vi "ValiseMarlin.vi"() -> ()   [LabVIEW 2017]
uses:
  Globals/VarGlobUIStopLoops.vi
  <resource>/objmgr/daqmx.rc
  DefDeType/WhichPath.ctl
  <vilib>/DAQmx/write.llb/DAQmx Write (Digital Bool 1Line 1Point).vi
  <vilib>/DAQmx/create/channels.llb/DAQmx Create Channel (DO-Digital Output).vi
  DefDeType/ClusterRefCtrl.ctl
panel:
  in  "Reprocess":bool
  in  "Next Test":u32
  out "AcqTime(s)":u16(slide) scale=0.0..1000.0
  out "Recording":bool
  in  "EnregistrerPtEtal":bool
  out "Projet":string
  in  "Essais réalisés":i32(listbox)
  out "Reload Config":bool
  out "EntreesTensions":dbl[][](graph)
  in  "ChangerConfig":bool
  out "iterationMonitoringLoop":i32
  out "iterationEventLoop":i32
  in  "Instruction":u8
  in  "Stop Enreg.":bool
  in  "Enregistrer":bool
  out "EtatValise":string
  out "AmplisPonts":dbl[][](graph)
  in  "Quitter":bool
  # "Commandes"
  # "Entrées Pont de Wheastone"
  # "Essais Réalisés"
  # "Entrées Tensions"
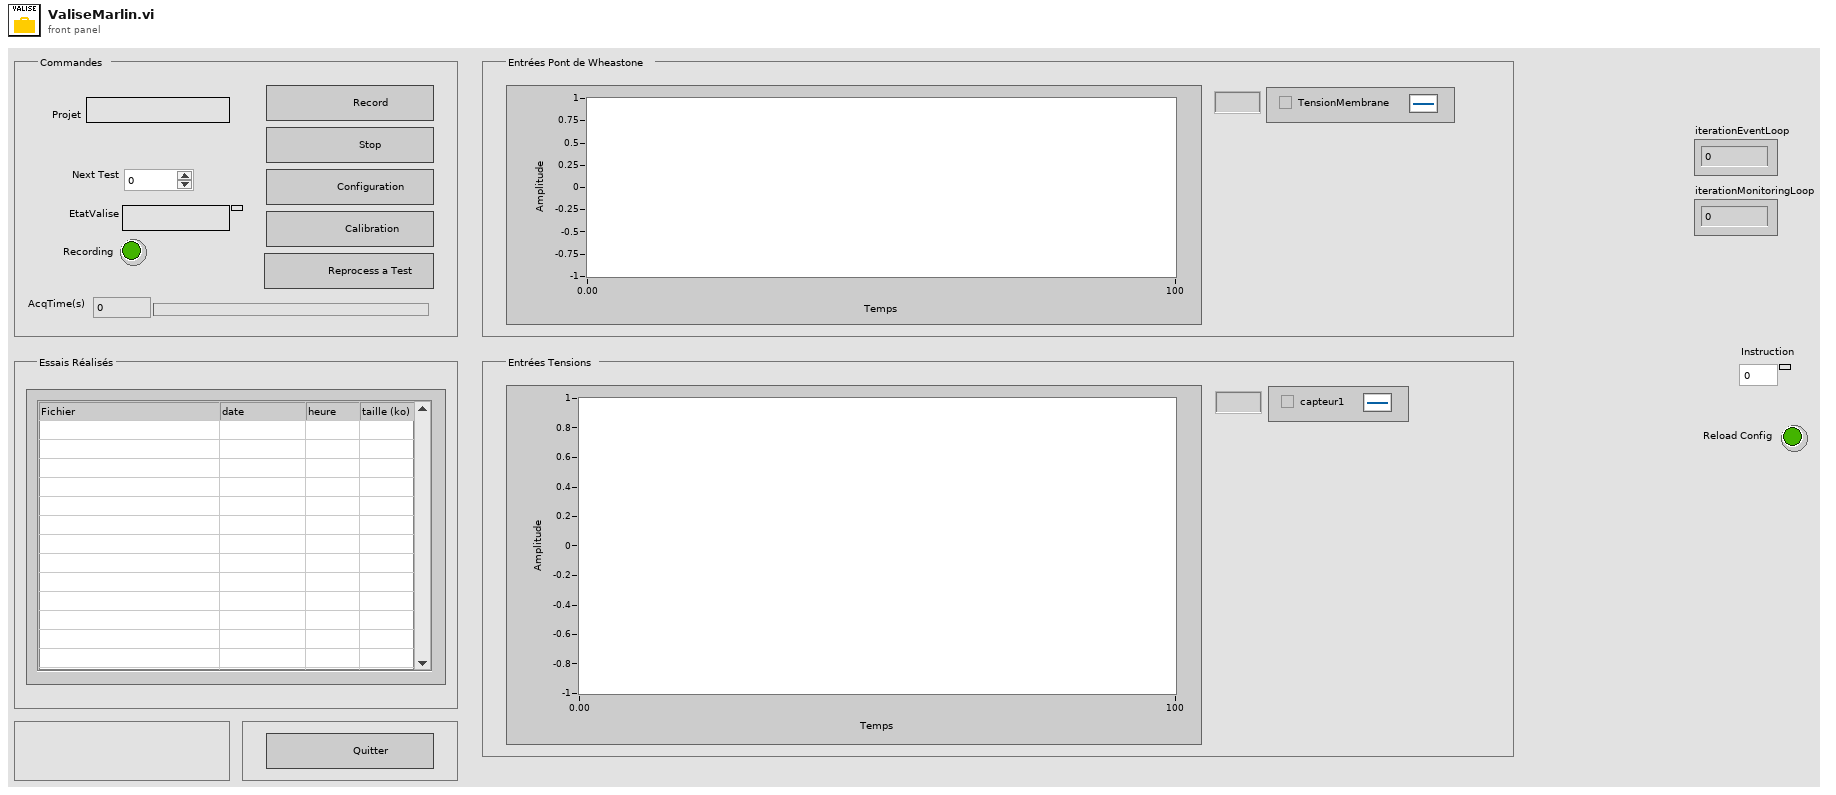
[diagram p1: front panel]
types:
  T1 = enum8{"Enabled", "Disabled", "Disabled and Grayed Out"}
  T2 = typedef "ClusterRefCtrl.ctl" = cluster{"Essais réalisés":refnum<vi>, "EnregistrerPtEtal":refnum<vi>, "ChangerConfig":refnum<vi>, "Enregistrer":refnum<vi>, "Reprocess":refnum<vi>}
  T3 = enum32{"Invalid", "Standard", "Closed", "Hidden", "Minimized", "Maximized"}
  T4 = cluster{"AcqTime(s)":refnum<vi>, "EntreesTensions":refnum<vi>, "AmplisPonts":refnum<vi>}
  T5 = typedef "ConfigTotale.ctl" = cluster{"VoltageChannels":T6, "WheastoneBridgeChannels":T7, "Configuration":T8}
  T6 = typedef "VoltageChannels.ctl" = cluster{"ChannelNames":string[], "Sensitivity(Unit/V)":dbl[], "AutoZero":bool[], "ChannelUnits":string[], "Offsets(Units)":dbl[], "Graph Num":u8[]}
  T7 = typedef "WBridgeChannels.ctl" = cluster{"ChannelNames":string[], "Sensitivity(Unit/V)":dbl[], "AutoZero":bool[], "ChannelUnits":string[], "Offsets(Units)":dbl[], "Graph Num":u8[]}
  T8 = typedef "Configuration.ctl" = cluster{"AcqSamplingRate(Hz)":u32, "AcqTime(s)":u32, "Trigger":bool, "NbVoltageChannels":u32, "NbWBridgeChannels":u32, "Qualisys":bool, "Hexapode":bool, "FinalSamplingRate(Hz)":u32, "QualisysDataType":enum16{"6DOF", "3DTracking", "6DOF + 3D"}, "Nortek":bool, "HBM":bool}
  T9 = typedef "WhichPath.ctl" = enum16{"DossierProjet", "Config", "Meas", "MeasPCI", "MeasCRIO1", "MeasCRIO2", "MeasQualisys", "MeasHBM", "MeasTDMS", "Fig", "Res"}
  T10 = typedef "MergeFileConfig.ctl" = cluster{"Test Num : ":u32, "Project :":string, "Qualisys file":path, "HBM file":path, "QualisysDataType":enum16{"6DOF", "3DTracking", "6DOF + 3D"}, "Qualisys":bool, "HBM":bool}
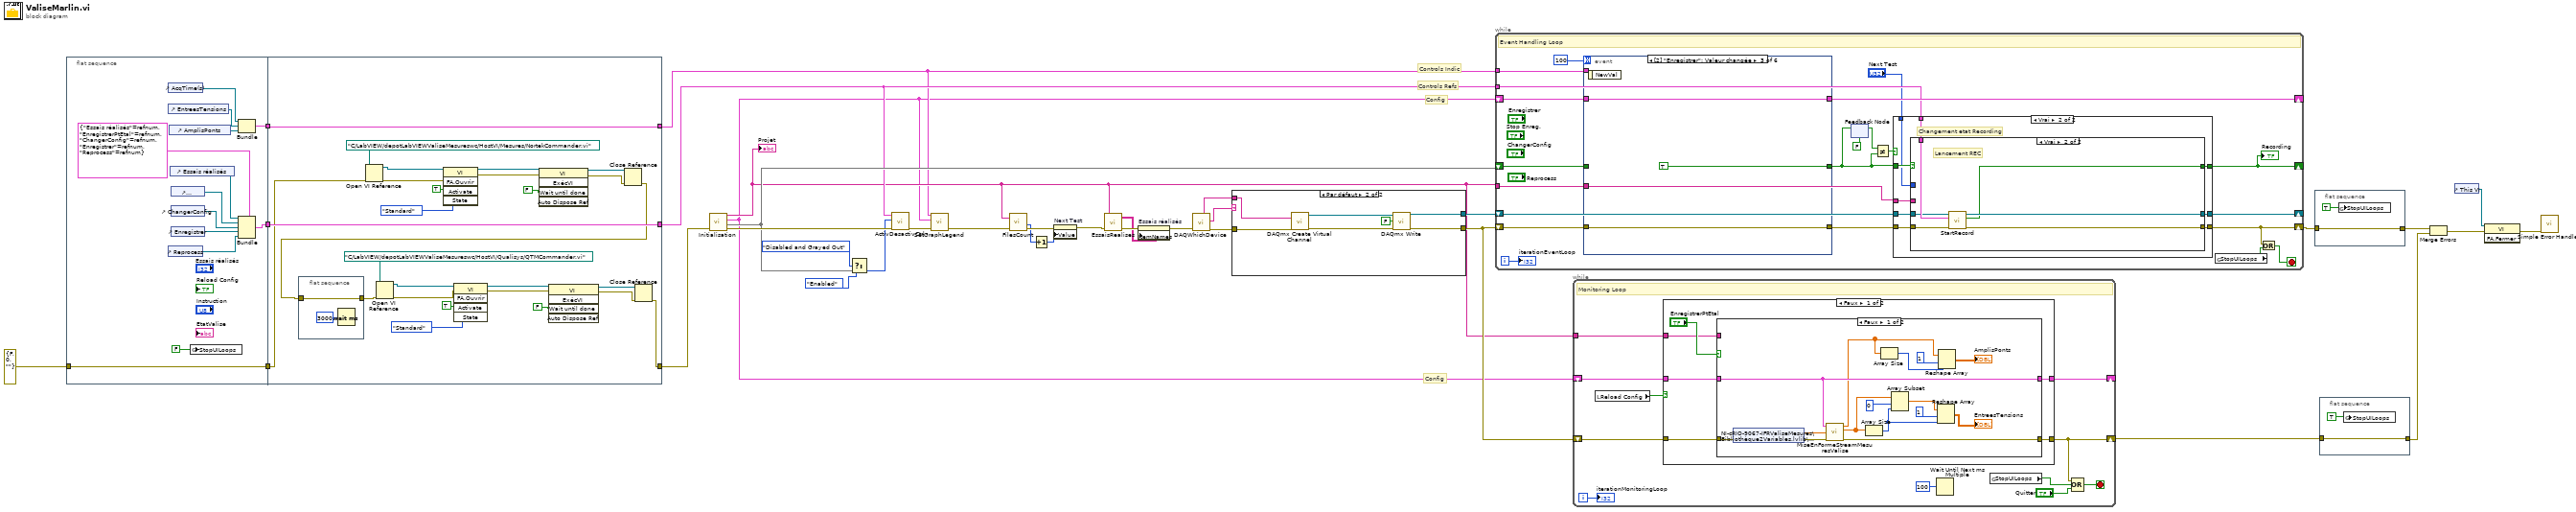
[diagram p0: block diagram]
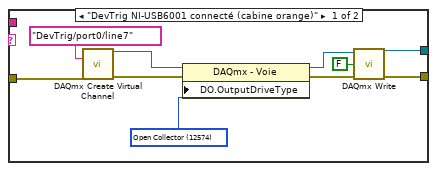
[diagram p2: hidden frame]
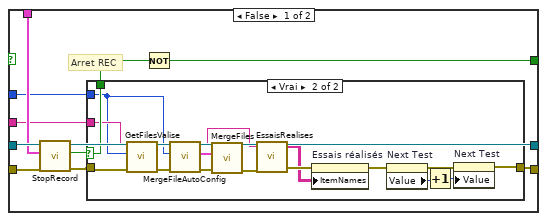
[diagram p4: hidden frame]
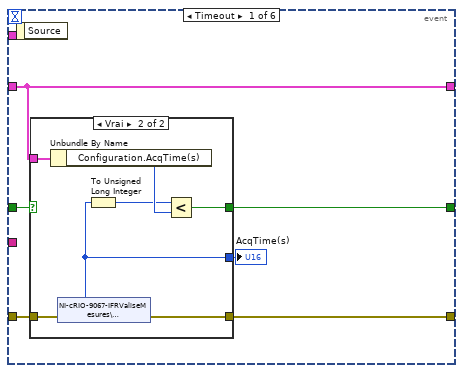
[diagram p6: hidden frame]
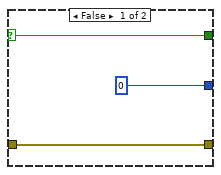
[diagram p7: hidden frame]
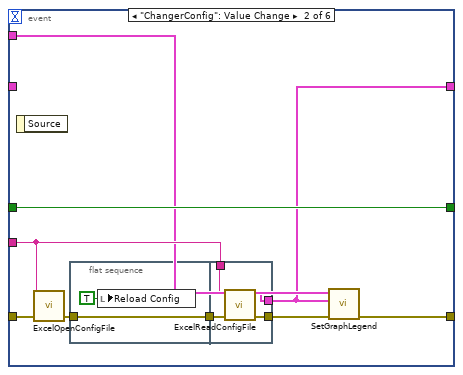
[diagram p8: hidden frame]
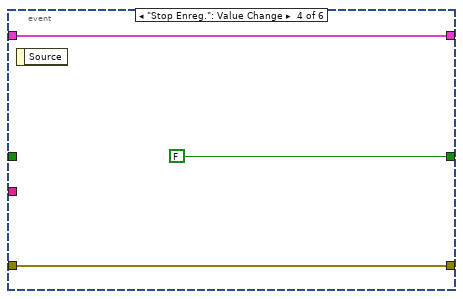
[diagram p9: hidden frame]
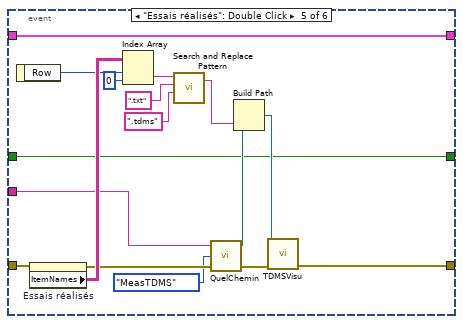
[diagram p10: hidden frame]
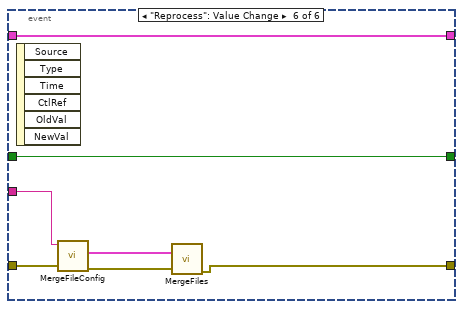
[diagram p11: hidden frame]
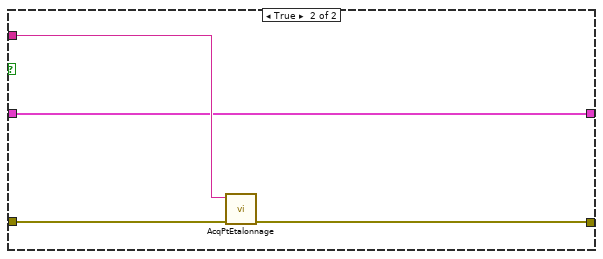
[diagram p12: hidden frame]
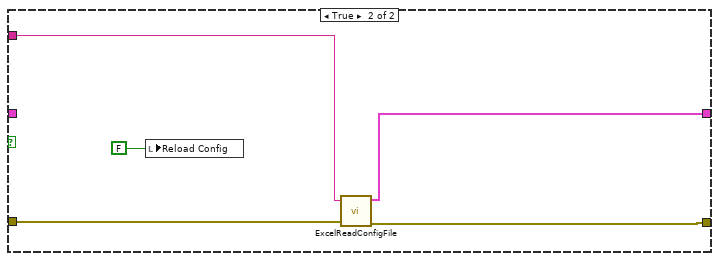
[diagram p13: hidden frame]
diagram:
  # "Controls Indic"
  # "Config"
  # "Config"
  # "Controls Refs"
  n1 = flat-sequence {
    tunnel: errorcluster {"status"=FALSE, "code"=0, "source"=""} ("entrée d'erreur (pas d'erreur)") -> [w47]
    tunnel: [w47] -> w3
    tunnel: [w42] -> w2
    tunnel: [w38] -> w1
    tunnel: [w73] -> w14
    tunnel: [w74] -> w21
    tunnel: [w51] -> w4
    tunnel: w3 -> [w52]
    tunnel: w2 -> [w74]
    tunnel: w1 -> [w73]
    frame #0 {
      n2 = control-ref of="EntreesTensions"() -> (w40:refnum<vi>)
      n3 = control-ref of="AcqTime(s)"() -> (w39:refnum<vi>)
      n4 = control-ref of="Reprocess"() -> (w36:refnum<vi>)
      n5 = control-ref of="AmplisPonts"() -> (w41:refnum<vi>)
      n6 = control-ref of="Essais réalisés"() -> (w43:refnum<vi>)
      n7 = control-ref of="EnregistrerPtEtal"() -> (w44:refnum<vi>)
      n8 = control-ref of="ChangerConfig"() -> (w45:refnum<vi>)
      n9 = control-ref of="Enregistrer"() -> (w46:refnum<vi>)
      n10 = global write "VarGlobUIStopLoops.vi" "StopUILoops"(FALSE ("StopUILoops")) -> ()
      n11 = Bundle("AcqTime(s)"=w39, "EntreesTensions"=w40, "AmplisPonts"=w41) -> (w38:T4)  [unwired: 1 in]
      n12 = Bundle(cluster=T2 {"Essais réalisés"=refnum, "EnregistrerPtEtal"=refnum, "ChangerConfig"=refnum, "Enregistrer"=refnum, "Reprocess"=refnum} ("Cluster"), "Essais réalisés"=w43, "EnregistrerPtEtal"=w44, "ChangerConfig"=w45, "Enregistrer"=w46, "Reprocess"=w36) -> (w42:T2)
    }
    frame #1 {
      n13 = flat-sequence {
        tunnel: w50 -> [w76]
        tunnel: [w76] -> w49
        frame #0 {
          n14 = Wait (ms)(milliseconds to wait=u32 3000) -> ()  [unwired: 1 out]
        }
      }
      n15 = Open VI Reference(vi path=path "C:/LabVIEW/depotLabVIEWValiseMesureswc/HostVI/Mesures/NortekCommander.vi", error in (no error)=w52) -> (vi reference=w54:refnum<vi>, error out=w55:errorcluster)  [unwired: 4 in]
      n16 = Open VI Reference(vi path=path "C:/LabVIEW/depotLabVIEWValiseMesureswc/HostVI/Qualisys/QTMCommander.vi", error in (no error)=w49) -> (vi reference=w71:refnum<vi>, error out=w70:errorcluster)  [unwired: 4 in]
      n17 = invoke class="VI" method="FA.Ouvrir"(reference=w54, error in=w55, "Activate"=TRUE ("Activate?"), "State"=T3."Standard") -> (reference out=w57:refnum<vi>, error out=w56:errorcluster)  [unwired: 1 in, 3 out]
      n18 = invoke class="VI" method="FA.Ouvrir"(reference=w71, error in=w70, "Activate"=TRUE ("Activate?"), "State"=T3."Standard") -> (reference out=w68:refnum<vi>, error out=w69:errorcluster)  [unwired: 1 in, 3 out]
      n19 = invoke class="VI" method="ExécVI"(reference=w57, error in=w56, "Wait until done"=FALSE ("Wait Until Done")) -> (reference out=w58:refnum<vi>, error out=w59:errorcluster)  [unwired: 2 in, 3 out]
      n20 = invoke class="VI" method="ExécVI"(reference=w68, error in=w69, "Wait until done"=FALSE ("Wait Until Done")) -> (reference out=w67:refnum<vi>, error out=w66:errorcluster)  [unwired: 2 in, 3 out]
      n21 = Close Reference(reference=w58, error in (no error)=w59) -> (error out=w50:errorcluster)
      n22 = Close Reference(reference=w67, error in (no error)=w66) -> (error out=w51:errorcluster)
    }
  }
  n23 = call "Initialisation.vi"("Error In"=w4) -> ("Error Out"=w26:errorcluster, 1:w25, "ConfigurationTotale"=w13:T5, "NomProjetOUT"=w20:string)  [unwired: 3 in]
  "Projet" <- w20
  n24 = Select(t=T1."Disabled and Grayed Out" ("Disabled"), s=w25, f=T1."Enabled" ("Disabled")) -> (s? t:f=w22:T1)
  n25 = call "ActivDesactivCtrl.vi"("error in (no error)"=w26, "Disabled"=w22, "Cluster"=w21) -> ("error out"=w15:errorcluster)  [unwired: 4 in]
  n26 = call "SetGraphLegend.vi"("error in (no error)"=w15, "ConfigTotale"=w13, "ClusterRefGraphs"=w14) -> ("error out"=w12:errorcluster)  [unwired: 4 in]
  n27 = call "FilesCount.vi"("NomProjet"=w20, "entrée d'erreur"=w12) -> ("NextTestNum"=w17:u32, "sortie d'erreur"=w19:errorcluster)  [unwired: 4 out]
  n28 = Increment(x=w17) -> (x+1=w16:u32)
  n29 = property on="Next Test" class="NumNb (strict)"(error in=w19, "Value"=w16) -> (error out=w18:errorcluster)  [unwired: 1 in, 1 out]
  n30 = call "EssaisRealises.vi"("entrée d'erreur (pas d'erreur)"=w18, "NomProjet"=w20) -> ("sortie d'erreur"=w30:errorcluster, "InfosFichiers"=w29:string[][])  [unwired: 2 in]
  n31 = property on="Essais réalisés" class="ListeMCol (strict)"(error in=w30, "ItemNames"=w29) -> (error out=w11:errorcluster)  [unwired: 1 in, 1 out]
  n32 = call "DAQWhichDevice.vi"("error in"=w11) -> ("error out"=w9:errorcluster, "Message"=w10:string, "DigitalInputFinAcq"=w8:tag)  [unwired: 1 in, 4 out]
  n33 = case shown="Par défaut" w10 {
    tunnel: [w79 w92] -> w28
    tunnel: [w78 w91] -> w27
    tunnel: w9 -> [w77 w90]
    tunnel: w8 -> [_ w87]
    frame "DevTrig NI-USB6001 connecté (cabine orange)" {
      w86 = 12574 items=["Active Drive"=12573, "Open Collector"=12574] ("DO.OutputDriveType")
      n34 = call-poly <vilib>:"DAQmx Create Virtual Channel.vi"("lines"=tag "DevTrig/port0/line7", "error in"=w77) -> ("task out"=w84:refnum<k21>, "error out"=w85:errorcluster)  [unwired: 12 in]
      n35 = property class="DAQmx - Voie"(reference=w84, error in=w85, "DO.OutputDriveType"=w86) -> (reference out=w81:refnum<k21>, error out=w80:errorcluster)
      n36 = call-poly <vilib>:"DAQmx Write.vi"("task/channels in"=w81, "data"=FALSE, "error in"=w80) -> ("task out"=w78:refnum<k21>, "error out"=w79:errorcluster)  [unwired: 10 in, 1 out]
    }
    frame Default {
      n37 = call-poly <vilib>:"DAQmx Create Virtual Channel.vi"("lines"=w87, "error in"=w90) -> ("task out"=w88:refnum<k21>, "error out"=w89:errorcluster)  [unwired: 12 in]
      n38 = call-poly <vilib>:"DAQmx Write.vi"("task/channels in"=w88, "data"=FALSE, "error in"=w89) -> ("task out"=w91:refnum<k21>, "error out"=w92:errorcluster)  [unwired: 10 in, 1 out]
    }
  }
  n39 = while {
    shift-right: [w102] -> w34
    shift-left: w28 -> [w113]
    tunnel: w20 -> [w95]
    shift-right: [w99] -> _
    shift-left: w25 -> [w109]
    tunnel: w21 -> [w101]
    shift-right: [w107] -> _
    shift-left: w13 -> [w108]
    shift-right: [w103] -> _
    shift-left: w27 -> [w94]
    tunnel: w14 -> [w96]
    i -> [w112]
    stop <- w110 stop-if-true
    # "Event Handling Loop"
    n40 = event shown="[2] \"Enregistrer\": Valeur changée" {
      selector: _ -> [_ _ _ _ _ _]
      dyn-events: _ -> [_ _ _ _ _ _]
      timeout: 100 -> [_ _ _ _ _ _]
      tunnel: w113 -> [w167 w187 w196 w199 w213 w223]
      tunnel: [w166 w179 w196 w199 w209 w219] -> w104
      tunnel: w95 -> [_ w185 _ _ w206 w220]
      tunnel: [w164 w186 TRUE ("recording?") FALSE ("recording?") w200 w217] -> w100
      tunnel: w109 -> [w168 w186 _ _ w200 w217]
      tunnel: w108 -> [w163 _ w194 w197 w201 w218]
      tunnel: [w163 w180 w194 w197 w201 w218] -> w107
      tunnel: w96 -> [_ w181 _ _ _ _]
      event Timeout {
        n41 = event-data() -> ()  [unwired: 1 in, 1 out]
        n42 = case shown="Vrai" w168 {
          selector: w168 -> [w169 _]
          tunnel: w167 -> [w171 w178]
          tunnel: [w171 w177] -> w166
          tunnel: w163 -> [_ w176]
          tunnel: [u16 0 ("UInt16") w172] -> w165
          tunnel: [w169 w173] -> w164
          frame False {
          }
          frame True {
            n43 = Unbundle By Name(w176) -> ("Configuration.AcqTime(s)"=w175:u32)
            n44 = shared-variable "NI-cRIO-9067-IFRValiseMesures\\Bibliothèque2Variables.lvlib\\AcqTime"(error in=w178) -> (w172:u16, error out=w177:errorcluster)
            n45 = To Unsigned Long Integer(number=w172) -> (unsigned 32bit integer=w174:u32)
            n46 = Less?(x=w174, y=w175) -> (x < y?=w173:bool)
          }
        }
        "AcqTime(s)" <- w165
      }
      event "ChangerConfig": Value Change {
        n47 = event-data() -> ()  [unwired: 1 in, 1 out]
        n48 = call "ExcelOpenConfigFile.vi"("error in (no error)"=w187, "NomProjet"=w185) -> ("sortie d'erreur"=w183:errorcluster)  [unwired: 2 in, 1 out]
        n49 = flat-sequence {
          tunnel: w183 -> [w189]
          tunnel: [w189] -> w184
          tunnel: [w192] -> w182
          tunnel: w184 -> [w193]
          tunnel: w185 -> [w191]
          tunnel: [w190] -> w180
          frame #0 {
            n50 = local write "Reload Config"(TRUE ("Reload Config")) -> ()
          }
          frame #1 {
            n51 = call "ExcelReadConfigFile.vi"("NomProjet"=w191, "error in (no error)"=w193) -> ("ConfigurationTotale"=w190:T5, "error out"=w192:errorcluster)  [unwired: 3 in]
          }
        }
        n52 = call "SetGraphLegend.vi"("error in (no error)"=w182, "ConfigTotale"=w180, "ClusterRefGraphs"=w181) -> ("error out"=w179:errorcluster)  [unwired: 4 in]
      }
      event "Enregistrer": Value Change {
        n53 = event-data() -> ()  [unwired: 1 in, 1 out]
      }
      event "Stop Enreg.": Value Change {
        n54 = event-data() -> ()  [unwired: 1 in, 1 out]
      }
      event "Essais réalisés": Double Click {
        n55 = event-data() -> ("Row"=w210:i32)  [unwired: 1 in]
        n56 = property on="Essais réalisés" class="ListeMCol (strict)"(error in=w213) -> (error out=w207:errorcluster, "ItemNames"=w212:string[][])  [unwired: 1 in, 1 out]
        n57 = Index Array(array=w212, index (row)=w210, index (col)=0 ("indice désactivé (col)")) -> (element=w214:string)
        n58 = call <vilib>:"Search and Replace Pattern.vi"("string"=w214, "regular expression (\"\")"=".txt" ("regular expression (\"\")"), "replace string (\"\")"=".tdms" ("replace string (\"\")")) -> ("result string"=w203:string)  [unwired: 2 in, 1 out]
        n59 = call "QuelChemin.vi"("Entrée d'erreur"=w207, "WhichPath?"=WhichPath."MeasTDMS", "NomProjet"=w206) -> ("Sortie d'erreur"=w208:errorcluster, "SurDisqueLocal"=w204:path)  [unwired: 1 out]
        n60 = Build Path(base path=w204, name or relative path=w203) -> (appended path=w202:path)
        n61 = call "TDMSVisu.vi"("error in (no error)"=w208, "file path"=w202) -> ("error out"=w209:errorcluster)  [unwired: 4 in, 1 out]
      }
      event "Reprocess": Value Change {
        n62 = event-data() -> ()  [unwired: 1 in, 6 out]
        n63 = call "MergeFileConfig.vi"("error in (no error)"=w223, "ProjetIN"=w220) -> ("error out"=w222:errorcluster, "MergeFileConfigOUT"=w221:T10)  [unwired: 3 in, 1 out]
        n64 = call "MergeFiles.vi"("Error In"=w222, "MergeFileConfigIN"=w221) -> ("sortie d'erreur"=w219:errorcluster)  [unwired: 5 in]
      }
    }
    n65 = feedback-in #1(w100) -> ()
    n66 = feedback #1(FALSE ("recording?")) -> (w106:bool)
    n67 = Not Equal?(x=w106, y=w100) -> (x != y?=w105:bool)
    n68 = case shown="Vrai" w105 {
      tunnel: [w116 w121] -> w102
      tunnel: w104 -> [w116 w125]
      tunnel: [w117 w120] -> w103
      tunnel: w94 -> [w117 w126]
      tunnel: w101 -> [_ w124]
      tunnel: w100 -> [w115 w123]
      tunnel: [w115 w122] -> w99
      tunnel: "Next Test" -> [_ w119]
      tunnel: w95 -> [_ w118]
      frame False {
      }
      frame True {
        # "Changement etat Recording"
        n69 = case shown="Vrai" w123 {
          tunnel: w126 -> [w136 w159]
          tunnel: w125 -> [w137 w162]
          tunnel: w124 -> [w135 w160]
          tunnel: [w133 w157] -> w122
          tunnel: [w130 w161] -> w121
          tunnel: [w134 w158] -> w120
          tunnel: w119 -> [w128 _]
          tunnel: w118 -> [w127 _]
          frame False {
            # "Arret REC"
            n70 = call "StopRecord.vi"("error in (no error)"=w137, "ClusterRefCtrlIN"=w135, "task/channels in"=w136) -> ("error out"=w131:errorcluster, "RecStopped"=w132:bool, "task out"=w134:refnum<k21>)  [unwired: 2 in]
            n71 = case shown="Vrai" w132 {
              selector: w132 -> [w138 w156]
              tunnel: w131 -> [w139 w147]
              tunnel: [w139 w151] -> w130
              tunnel: [w138 w156] -> w129
              tunnel: w128 -> [_ w144]
              tunnel: w127 -> [_ w148]
              frame False {
              }
              frame True {
                n72 = call "GetFilesValise.vi"("error in (no error)"=w147, "Test Num :"=w144, "Project :"=w148) -> ("error out"=w145:errorcluster, "NomProjetOut"=w146:string)  [unwired: 3 in]
                n73 = call "MergeFileAutoConfig.vi"("error in (no error)"=w145, "test num"=w144, "ProjetIN"=w146) -> ("error out"=w142:errorcluster, "MergeFileConfigOUT"=w143:T10, "ProjetOUT"=w140:string)  [unwired: 2 in]
                n74 = call "MergeFiles.vi"("Error In"=w142, "MergeFileConfigIN"=w143) -> ("sortie d'erreur"=w141:errorcluster)  [unwired: 5 in]
                n75 = call "EssaisRealises.vi"("entrée d'erreur (pas d'erreur)"=w141, "NomProjet"=w140) -> ("sortie d'erreur"=w155:errorcluster, "InfosFichiers"=w154:string[][])  [unwired: 2 in]
                n76 = property on="Essais réalisés" class="ListeMCol (strict)"(error in=w155, "ItemNames"=w154) -> (error out=w153:errorcluster)  [unwired: 1 in, 1 out]
                n77 = property on="Next Test" class="NumNb (strict)"(error in=w153) -> (error out=w152:errorcluster, "Value"=w150:u32)  [unwired: 1 in, 1 out]
                n78 = Increment(x=w150) -> (x+1=w149:u32)
                n79 = property on="Next Test" class="NumNb (strict)"(error in=w152, "Value"=w149) -> (error out=w151:errorcluster)  [unwired: 1 in, 1 out]
              }
            }
            n80 = Not(x=w129) -> (.not. x?=w133:bool)
          }
          frame True {
            # "Lancement REC"
            n81 = call "StartRecord.vi"("error in (no error)"=w162, "ClusterRefCtrlIN"=w160, "task/channels in"=w159) -> ("error out"=w161:errorcluster, "RecStarted"=w157:bool, "task out"=w158:refnum<k21>)  [unwired: 2 in]
          }
        }
      }
    }
    "Recording" <- w99
    n82 = global read "VarGlobUIStopLoops.vi" "StopUILoops"() -> (w111:bool)
    n83 = Or(x=w102, y=w111) -> (x .or. y?=w110:bool)
    "iterationEventLoop" <- w112
  }
  n84 = while {
    shift-right: [w228] -> w33
    shift-left: w28 -> [w233]
    shift-right: [w225] -> _
    shift-left: w13 -> [w227]
    tunnel: w20 -> [w224]
    i -> [w232]
    stop <- w231 stop-if-true
    # "Monitoring Loop"
    n85 = local read "Reload Config"() -> (w226:bool)
    n86 = case shown="Faux" w226 {
      tunnel: w233 -> [w240 w264]
      tunnel: [w239 w263] -> w228
      tunnel: w227 -> [w238 _]
      tunnel: [w237 w262] -> w225
      tunnel: w224 -> [w235 w261]
      frame False {
        n87 = case shown="Faux" "EnregistrerPtEtal" {
          tunnel: w240 -> [w253 w258]
          tunnel: [w247 w257] -> w239
          tunnel: w238 -> [w245 w256]
          tunnel: [w245 w256] -> w237
          tunnel: w235 -> [_ w259]
          frame False {
            n88 = shared-variable "NI-cRIO-9067-IFRValiseMesures\\Bibliothèque2Variables.lvlib\\ApercuMesures"(error in=w253) -> (w246:dbl[], error out=w248:errorcluster)
            n89 = call "MiseEnFormeStreamMesuresValise.vi"("Error In"=w248, "MesuresBrutesValise"=w246, "ConfigTotale"=w245) -> ("Error Out"=w247:errorcluster, "VoltageChannels1(0to15)"=w242:dbl[], "WBridgeChannels"=w244:dbl[])  [unwired: 2 in]
            n90 = Array Size(array=w242) -> (size(s)=w241:i32)
            n91 = Array Size(array=w244) -> (size(s)=w243:i32)
            n92 = Array Subset(array=w242, index=0 ("indice"), length=w241) -> (w249:dbl[])
            n93 = Reshape Array(w249, 1 ("taille de la dimension"), w241) -> (→"EntreesTensions":dbl[][])
            n94 = Reshape Array(w244, 1 ("taille de la dimension"), w243) -> (→"AmplisPonts":dbl[][])
          }
          frame True {
            n95 = call "AcqPtEtalonnage.vi"("entrée d'erreur"=w258, "Projet"=w259) -> ("sortie d'erreur"=w257:errorcluster)  [unwired: 5 in]
          }
        }
      }
      frame True {
        n96 = local write "Reload Config"(FALSE ("Reload Config")) -> ()
        n97 = call "ExcelReadConfigFile.vi"("NomProjet"=w261, "error in (no error)"=w264) -> ("ConfigurationTotale"=w262:T5, "error out"=w263:errorcluster)  [unwired: 3 in]
      }
    }
    n98 = Wait Until Next ms Multiple(millisecond multiple=u32 100 ("n millisecondes")) -> ()  [unwired: 1 out]
    n99 = global read "VarGlobUIStopLoops.vi" "StopUILoops"() -> (w230:bool)
    n100 = Compound Arithmetic op=OR ("Opérateur arithmétique")(w228, w230, "Quitter") -> (w231:bool)
    "iterationMonitoringLoop" <- w232
  }
  n101 = flat-sequence {
    tunnel: w34 -> [w265]
    tunnel: [w265] -> w32
    frame #0 {
      n102 = global write "VarGlobUIStopLoops.vi" "StopUILoops"(TRUE ("StopUILoops")) -> ()
    }
  }
  n103 = flat-sequence {
    tunnel: w33 -> [w267]
    tunnel: [w267] -> w31
    frame #0 {
      n104 = global write "VarGlobUIStopLoops.vi" "StopUILoops"(TRUE ("StopUILoops")) -> ()
    }
  }
  n105 = Merge Errors(w32, w31) -> (w5:errorcluster)
  n106 = control-ref of="This VI"() -> (w7:refnum<vi>)
  n107 = invoke class="VI" method="FA.Fermer"(reference=w7, error in=w5) -> (error out=w6:errorcluster)  [unwired: 1 in, 2 out]
  n108 = call <vilib>:"Simple Error Handler.vi"("error in (no error)"=w6) -> ()  [unwired: 4 in, 5 out]
